vi "BRig_RT_timeLoop_Exp.vi"(7 "input_error":errorcluster, 8 "input_Threshold_reset":bool, 9 "input_Threshold":bool, 10 "input_timestamp":timestamp, 11 "input_state":T1=enum."setSettings_Laser") -> (1 "output_Threshold":bool, 2 "output_duration":dbl, 5 "error out":errorcluster)   [LabVIEW 2014]
uses:
  myRIO_BRig_RT__Case_Exp_stateList.ctl
panel:
  out "Numeric":dbl
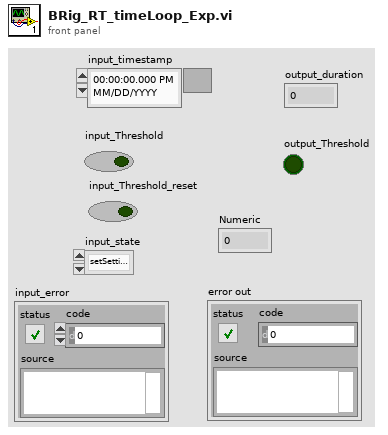
[diagram p1: front panel]
types:
  T1 = typedef "myRIO_BRig_RT__Case_Exp_stateList.ctl" = enum16{"Start1", "Start2", "Start3", "saveSettings1", "saveSettings2", "saveSettings3", "saveSettings4", "saveSettings_LC_ENL_l1", "saveSettings_LC_ENL_l2", "saveSettings_LC_Cue_l1", "saveSettings_LC_Cue_l2", "saveSettings6_LC_l1_Other", "SaveSettings6_LC_l2_Other", "setSettings_Audio", "setSettings_Laser", "initBlock_pre", "initBlock", "initBlock2", "initBlock_post", "initTrial_pre", "initTrial", "initTrial2", "initTrial3", "initTrial4", "initTrial_LC_ENL1", "initTrial_LC_Cue1", "initTrial_LC_Cue1_2", "initTrial_LC_Sel", "initTrial_post", "ENL1_pre", "ENL1", "ENL1_post", "ENL1Penalty_pre", "ENL1Penalty", "ENL2_pre", "ENL2", "ENL2Penalty_pre", "ENL2Penalty", "Cue1_pre", "Cue1", "Cue1_post", "Cue1Penalty_pre", "Cue1Penalty", "Cue2_pre", "Cue2", "Cue2Penalty_pre", "Cue2Penalty", "Selection_pre", "Selection", "Select_post", "SelectReward_pre", "SelectReward", "SelectRewardPost_pre", "SelectRewardPost", "SelectWrong_pre", "SelectWrong", "SelectWrong_post", "SelectTimeout_pre", "SelectTimeout", "SelectTimeout_post", "endTrial_pre", "endTrial1", "endTrial2", "endTrial3", "endTrial_post", "endBlock_pre", "endBlock", "endBlock_post", "endExp", "commConnect", "commUpload_pre", "commUpload_dataBlock", "commUpload_dataCurrent", "commUpload_dataExp", "commUpload_dataLC", "commUpload_dataTrial", "commUpload_post", "saveData_pre", "saveData_dataBlock", "saveData_dataCurrent", "saveData_dataExp", "saveData_dataLC", "saveData_dataTrial", "saveData_post", "empty_endBlock1", "empty_endBlock2", "empty_endTrial1", "empty_endTrial2", "empty_endTrial3", "empty_endTrial4", "empty_endTrial5", "dummyState", "dummyState_endBlock", "FreeReward_pre", "FreeReward", "FreeRewardPost_pre", "FreeRewardPost"}
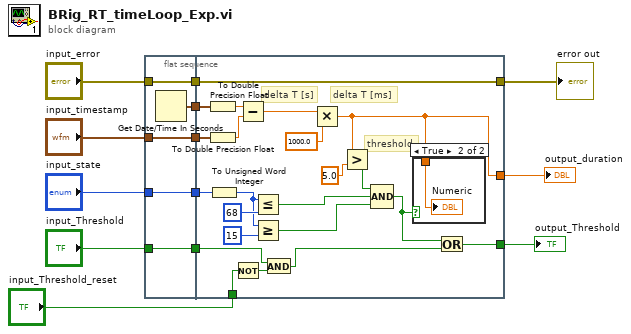
[diagram p0: block diagram]
diagram:
  n1 = flat-sequence {
    tunnel: "input_error" -> [w18]
    tunnel: "input_timestamp" -> [w16]
    tunnel: [w18] -> w13
    tunnel: [w17] -> w12
    tunnel: [w16] -> w11
    tunnel: "input_Threshold" -> [w15]
    tunnel: [w15] -> w10
    tunnel: [w14] -> w3
    tunnel: "input_state" -> [w14]
    tunnel: [w40] -> w8
    tunnel: w13 -> [w40]
    tunnel: w12 -> [w39]
    tunnel: w11 -> [w37]
    tunnel: w10 -> [w23]
    tunnel: [w32] -> w6
    tunnel: [w20] -> w5
    tunnel: w3 -> [w31]
    tunnel: "input_Threshold_reset" -> [w25]
    frame #0 {
      n2 = Get Date/Time In Seconds() -> (seconds since 1Jan1904=w17:timestamp)
    }
    frame #1 {
      # "threshold"
      # "delta T [ms]"
      # "delta T [s]"
      n3 = To Double Precision Float(number=w39) -> (double precision float=w38:dbl)
      n4 = To Double Precision Float(number=w37) -> (double precision float=w36:dbl)
      n5 = To Unsigned Word Integer(number=w31) -> (unsigned 16bit integer=w28:u16)
      n6 = Not(x=w25) -> (.not. x?=w24:bool)
      n7 = Subtract(x=w38, y=w36) -> (x-y=w35:dbl)
      n8 = Less Or Equal?(x=w28, y=u16 68) -> (x <= y?=w30:bool)
      n9 = Greater Or Equal?(x=w28, y=u16 15) -> (x >= y?=w26:bool)
      n10 = And(x=w23, y=w24) -> (x .and. y?=w22:bool)
      n11 = Multiply(x=w35, y=1000.0) -> (x*y=w20:dbl)
      n12 = Greater?(x=w20, y=5.0) -> (0:w21:bool)
      n13 = Compound Arithmetic op=AND(w21, w30, w26) -> (w19:bool)
      n14 = case shown="True" w19 {
        tunnel: w20 -> [_ w41]
        frame False {
        }
        frame True {
          "Numeric" <- w41
        }
      }
      n15 = Or(x=w19, y=w22) -> (x .or. y?=w32:bool)
    }
  }
  "error out" <- w8
  "output_Threshold" <- w6
  "output_duration" <- w5
